vi "Undeploy SV Libraries.vi"(8 "error in (no error)":errorcluster, 11 "SV B-M in":refnum<class "SV B-M (Host).lvclass">) -> (0 "error out":errorcluster, 3 "SV B-M out":refnum<class "SV B-M (Host).lvclass">)   [LabVIEW 2015, in "SV B-M (Host).lvclass"]
doc: "Undeploy all shared variable libraries used in this test."
uses:
  SV B-M (Host).lvclass
  SV B-M (Host).lvclass/SV B-M (Host).ctl
  Listbox - In Progress.vi
  Listbox - Complete.vi
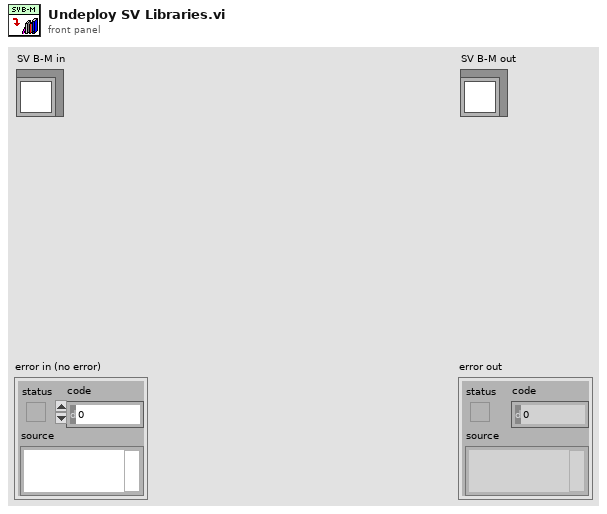
[diagram p1: front panel]
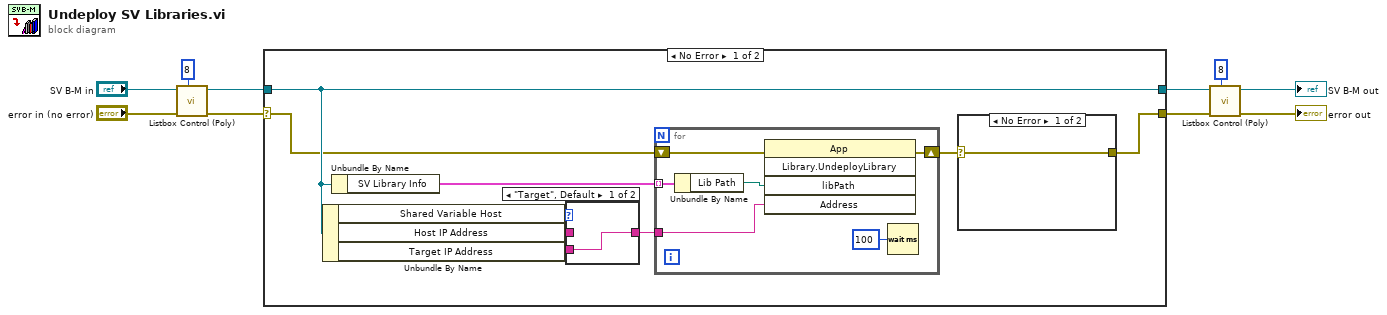
[diagram p0: block diagram]
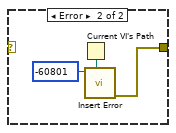
[diagram p2: hidden frame]
diagram:
  n1 = call-poly "Listbox Control (Poly).vi"("Row to Update"=8, "error in (no error)"="error in (no error)", "SV B-M In"="SV B-M in") -> ("error out"=w1:errorcluster, "SV B-M Out"=w8:refnum<class "SV B-M (Host).lvclass">)  [unwired: 7 in]
  n2 = case shown="No Error" w1 {
    selector: w1 -> [w13 w32]
    tunnel: [w16 w33] -> w4
    tunnel: w8 -> [w16 w33]
    tunnel: [w11 w32] -> w5
    frame No Error {
      n3 = Unbundle By Name(w16) -> ("Shared Variable Host"=w19:enum16{"Target", "Host"}, "Host IP Address"=w18:string, "Target IP Address"=w17:string)
      n4 = Unbundle By Name(w16) -> ("SV Library Info"=w15:cluster{"Lib Path":path, "Lib Size":u16}[])
      n5 = case shown="\"Target\", Default" w19 {
        tunnel: w18 -> [_ w31]
        tunnel: w17 -> [w30 _]
        tunnel: [w30 w31] -> w14
        frame "Target", Default {
        }
        frame "Host" {
        }
      }
      n6 = for {
        tunnel: w15 -> [w29] mode=indexing
        tunnel: w14 -> [w26]
        shift-right: [w24] -> w12
        shift-left: w13 -> [w27]
        n7 = Unbundle By Name(w29) -> ("Lib Path"=w28:path)
        n8 = invoke class="App" method="Library.UndeployLibrary"(error in=w27, "libPath"=w28, "Address"=w26) -> (error out=w24:errorcluster)  [unwired: 2 in, 4 out]
        n9 = Wait (ms)(milliseconds to wait=u32 100) -> ()  [unwired: 1 out]
      }
      n10 = case shown="No Error" w12 {
        selector: w12 -> [w20 _]
        tunnel: [w20 w21] -> w11
        frame No Error {
        }
        frame Error {
          n11 = Current VI's Path() -> (path=w22:path)
          n12 = call "Insert Error.vi"("VI Path"=w22, "Error Code"=-60801) -> ("error out"=w21:errorcluster)  [unwired: 9 in]
        }
      }
    }
    frame Error {
    }
  }
  n13 = call-poly "Listbox Control (Poly).vi"("Row to Update"=8, "error in (no error)"=w5, "SV B-M In"=w4) -> ("error out"=→"error out":errorcluster, "SV B-M Out"=→"SV B-M out":refnum<class "SV B-M (Host).lvclass">)  [unwired: 7 in]
